vi "subimage.vi"(6 "Ysz/2":i32, 7 "Xsz/2":i32, 9 "Yc":i32, 10 "Xc":i32, 11 "ImgData":sgl[][](array[numeric])) -> (3 "SubImg":sgl[][](array[numeric]))   [LabVIEW 2019]
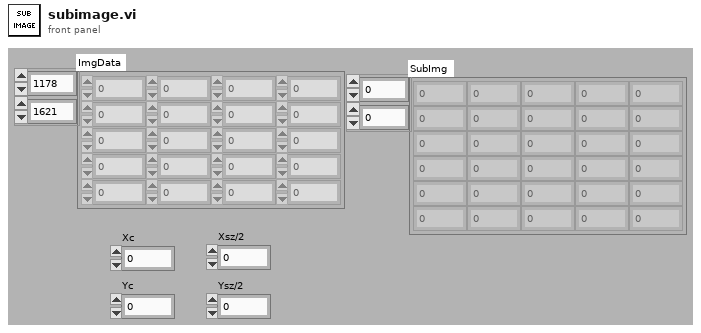
[diagram p1: front panel]
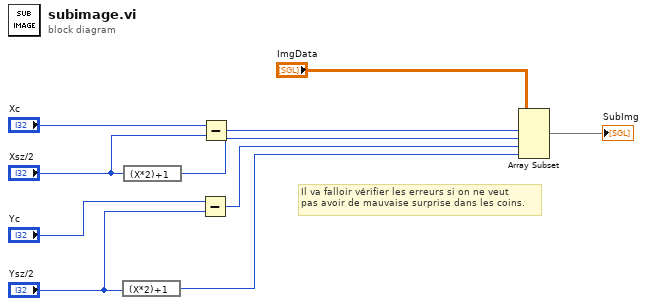
[diagram p0: block diagram]
diagram:
  # "Il va falloir vérifier les erreurs si on ne veut\npas avoir de mauvaise surprise dans les coins."
  n1 = expression code="(X*2)+1"("Ysz/2") -> (w2:i32)
  n2 = expression code="(X*2)+1"("Xsz/2") -> (w5:i32)
  n3 = Subtract(x="Yc", y="Ysz/2") -> (x-y=w10:i32)
  n4 = Subtract(x="Xc", y="Xsz/2") -> (x-y=w9:i32)
  n5 = Array Subset(array="ImgData", index (row)=w9, length (row)=w5, index (col)=w10, length (col)=w2) -> (→"SubImg":sgl[][])
